vi "AFT Linear Prediction.vi"   [LabVIEW 2017, in "NI_AdaptiveFilter.lvlib"]
doc: "Performs adaptive linear prediction by estimating the autoregressive (AR) model of an input signal. Wire data to the <B>signal</B> input to determine the polymorphic instance to use or manually select the instance."
uses:
  <vilib>/addons/Adaptive Filters/NI_AdaptiveFilter.lvlib
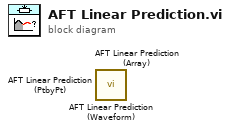
[diagram p0: block diagram]
diagram:
  n1 = call <vilib>:"AFT Linear Prediction (Waveform).vi"() -> ()  [unwired: 8 in, 4 out]
  n2 = call <vilib>:"AFT Linear Prediction (Array).vi"() -> ()  [unwired: 8 in, 4 out]
  n3 = call <vilib>:"AFT Linear Prediction (PtbyPt).vi"() -> ()  [unwired: 8 in, 4 out]
